vi "find instance.vi"(8 "error in":errorcluster, 10 "ID":string, 11 "memory hierarchy":T1) -> (0 "error out":errorcluster, 3 "configuration":refnum<class "NISE_CEF_serializable configuration.lvclass">)   [LabVIEW 2013, in "NISE_CEF_TreeSerializer.lvlib"]
uses:
  NISE_CEF_TreeSerializer.lvlib
  memory hierarchy.ctl
  hierarchy element.ctl
  serializable configuration/NISE_CEF_serializable configuration.lvclass
  NISE_CEF_TreeControl.lvlib
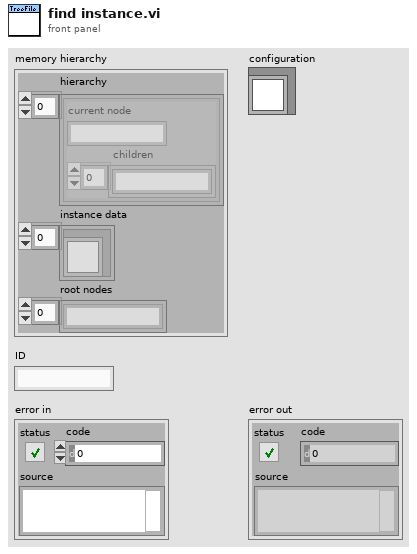
[diagram p1: front panel]
types:
  T1 = typedef "NISE_CEF_TreeSerializer.lvlib/memory hierarchy.ctl" = cluster{"hierarchy":T2[], "instance data":refnum<class "NISE_CEF_serializable configuration.lvclass">[], "root nodes":string[]}
  T2 = typedef "NISE_CEF_TreeSerializer.lvlib/hierarchy element.ctl" = cluster{"current node":string, "children":string[]}
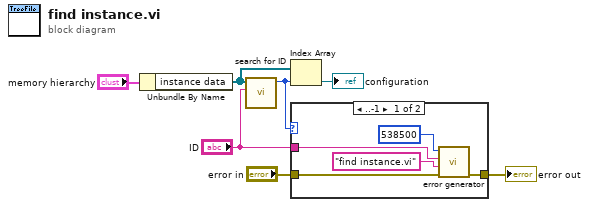
[diagram p0: block diagram]
diagram:
  n1 = Unbundle By Name("memory hierarchy") -> ("instance data"=w6:refnum<class "NISE_CEF_serializable configuration.lvclass">[])
  n2 = call "search for ID.vi"("instance id"="ID", "instance data"=w6) -> ("index"=w4:i32)  [unwired: 9 in]
  n3 = Index Array(array=w6, index=w4) -> (element=→"configuration":refnum<class "NISE_CEF_serializable configuration.lvclass">)
  n4 = case shown="..-1" w4 {
    tunnel: [w11 w13] -> w3
    tunnel: "error in" -> [w12 w13]
    tunnel: "ID" -> [w9 _]
    frame ..-1 {
      n5 = call "error generator.vi"("error in"=w12, "source"="find instance.vi", "append error message"=w9, "error code (0)"=538500) -> ("error out"=w11:errorcluster)  [unwired: 5 in]
    }
    frame 0.. {
    }
  }
  "error out" <- w3
